vi "WriteConfig.vi"(8 "error in (no error)":errorcluster, 10 "Config":variant, 11 "RoomAlert in":refnum<class "RoomAlert.lvclass">) -> (0 "error out":errorcluster, 3 "RoomAlert out":refnum<class "RoomAlert.lvclass">)   [LabVIEW 2018, in "SensorPlugins.lvlib" / "RoomAlert.lvclass"]
uses:
  RoomAlert.lvclass
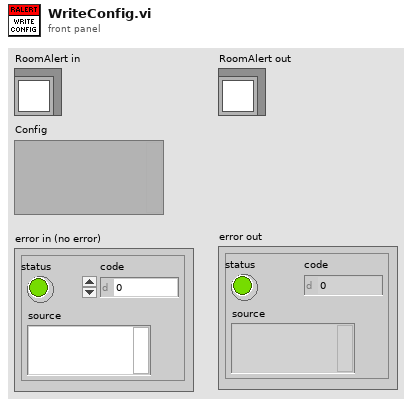
[diagram p1: front panel]
types:
  T1 = typedef "SensorPlugins.lvlib/RoomAlert.lvclass/MeasurementControls.ctl" = cluster{"Measurement RefreshTime (ms)":u32, "Measurement Name":string, "Timeout(ms)":i32}
  T2 = typedef "SensorPlugins.lvlib/RoomAlert.lvclass/RoomAlertControls.ctl" = cluster{"Connected?":bool, "IP Address of SNMP Device":string, "Port (161)":u16, "Community Name":string, "Measurements To Read Array":u16[], "Update Light \nTower?":bool, "LightTower":cluster{"Red":bool, "Amber":bool, "Green":bool, "Audio":bool}}[]
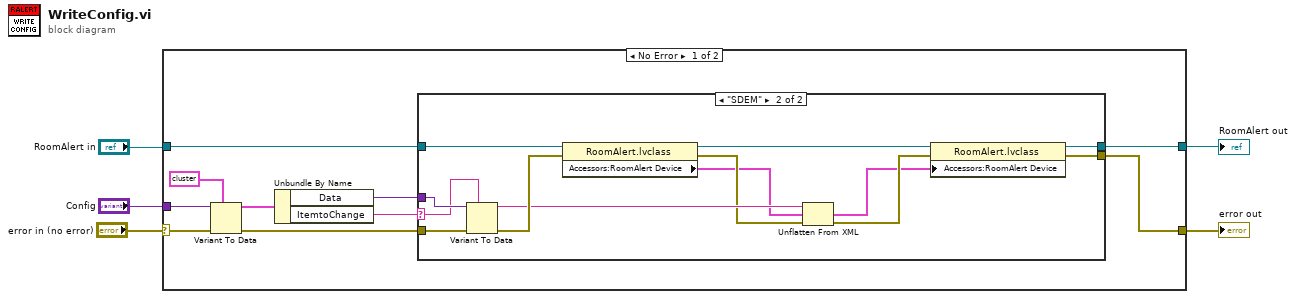
[diagram p0: block diagram]
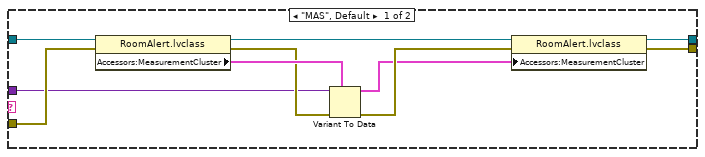
[diagram p2: hidden frame]
diagram:
  n1 = case shown="No Error" "error in (no error)" {
    selector: "error in (no error)" -> [w13 w40]
    tunnel: [w7 w40] -> w1
    tunnel: "RoomAlert in" -> [w15 w39]
    tunnel: [w6 w39] -> w2
    tunnel: "Config" -> [w14 _]
    frame No Error {
      n2 = Variant To Data(error in=w13, type=cluster{"Data":variant, "ItemtoChange":string} {"Data"=variant, "ItemtoChange"=""}, Variant=w14) -> (data=w10:cluster{"Data":variant, "ItemtoChange":string}, error out=w12:errorcluster)
      n3 = Unbundle By Name(w10) -> ("Data"=w9:variant, "ItemtoChange"=w8:string)
      n4 = case shown="\"SDEM\"" w8 {
        selector: w8 -> [_ w31]
        tunnel: w15 -> [w25 w38]
        tunnel: [w23 w36] -> w6
        tunnel: [w22 w35] -> w7
        tunnel: w12 -> [w21 w33]
        tunnel: w9 -> [w18 w34]
        frame "MAS", Default {
          n5 = property class="RoomAlert.lvclass"(reference=w25, error in=w21) -> (reference out=w24:refnum<class "RoomAlert.lvclass">, error out=w19:errorcluster, "Accessors:MeasurementCluster"=w20:T1)
          n6 = Variant To Data(error in=w19, type=w20, Variant=w18) -> (data=w16:T1, error out=w17:errorcluster)
          n7 = property class="RoomAlert.lvclass"(reference=w24, error in=w17, "Accessors:MeasurementCluster"=w16) -> (reference out=w23:refnum<class "RoomAlert.lvclass">, error out=w22:errorcluster)
        }
        frame "SDEM" {
          n8 = Variant To Data(error in=w33, type=w31, Variant=w34) -> (data=w30:string, error out=w32:errorcluster)
          n9 = property class="RoomAlert.lvclass"(reference=w38, error in=w32) -> (reference out=w37:refnum<class "RoomAlert.lvclass">, error out=w29:errorcluster, "Accessors:RoomAlert Device"=w28:T2)
          n10 = Unflatten From XML(xml string=w30, type=w28, error in (no error)=w29) -> (value=w26:T2, error out=w27:errorcluster)
          n11 = property class="RoomAlert.lvclass"(reference=w37, error in=w27, "Accessors:RoomAlert Device"=w26) -> (reference out=w36:refnum<class "RoomAlert.lvclass">, error out=w35:errorcluster)
        }
      }
    }
    frame Error {
    }
  }
  "error out" <- w1
  "RoomAlert out" <- w2
